vi "RD_3_data(COGNEX).vi"(6 "index (row)":i32, 7 "Array":dbl[](array[numeric]), 9 "Data array 2":sgl[][](array[numeric]), 11 "Data array":sgl[][](array[numeric])) -> (1 "output array 2":sgl[][](array[numeric]), 3 "output array":sgl[][](array[numeric]))   [LabVIEW 2019]
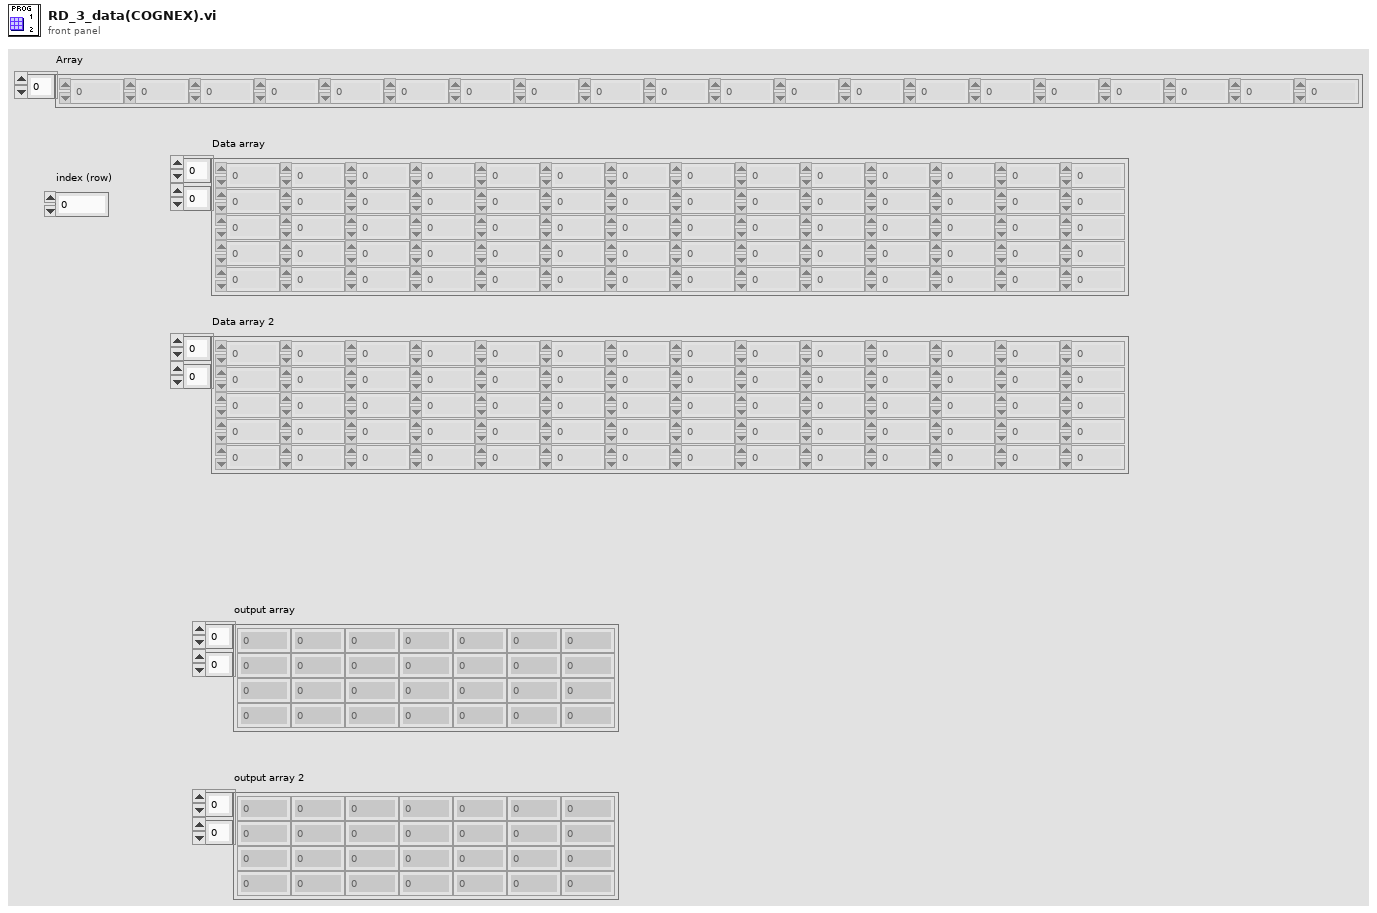
[diagram p1: front panel]
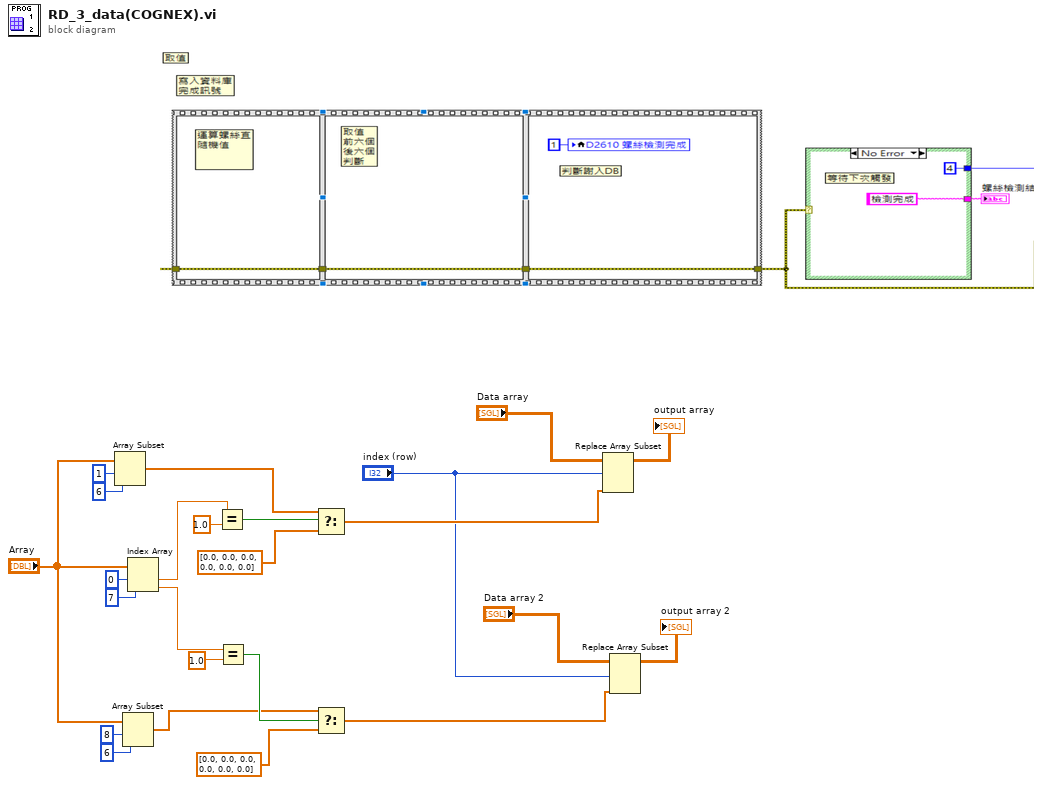
[diagram p0: block diagram]
diagram:
  n1 = Array Subset(array="Array", index=1, length=6) -> (w8:dbl[])
  n2 = Array Subset(array="Array", index=8, length=6) -> (w4:dbl[])
  n3 = Index Array(array="Array", index #1=0 ("index"), index #2=7 ("index")) -> (element #1=w13:dbl, element #2=w10:dbl)
  n4 = Equal?(x=w13, y=1.0) -> (x = y?=w9:bool)
  n5 = Equal?(x=w10, y=1.0) -> (x = y?=w5:bool)
  n6 = Select(t=w8, s=w9, f=dbl[] [0.0, 0.0, 0.0, 0.0, 0.0, 0.0]) -> (s? t:f=w6:dbl[])
  n7 = Select(t=w4, s=w5, f=dbl[] [0.0, 0.0, 0.0, 0.0, 0.0, 0.0]) -> (s? t:f=w1:dbl[])
  n8 = Replace Array Subset(array="Data array", new element=w6, index (row)="index (row)") -> (→"output array":sgl[][])  [unwired: 1 in]
  n9 = Replace Array Subset(array="Data array 2", new element=w1, index (row)="index (row)") -> (→"output array 2":sgl[][])  [unwired: 1 in]
